vi "FPGA Target Approach RetractionA2copyAidan.vi"() -> ()   [LabVIEW 2012]
uses:
  <vilib>/rvi/FXPMathLib/basic elements/FxpIntAccumulator/subVIs/nifxpmath_IntAccumulator_SimConfig.ctl
  <vilib>/rvi/eio/common/nirviEmuTemplateMethod_errors.vi
  <vilib>/rvi/FXPMathLib/basic elements/FxpIntAccumulator/simVIs/DllFxpIntAccumulator_sub.vi
  <vilib>/rvi/interface/RandomDataEmulation/nirviRandomDataFPGAFIFO.vi
  <vilib>/rvi/interface/RandomDataEmulation/niFpgaRandomDataHandleErrors.vi
  <vilib>/rvi/Emulation/niFpgaSctlEmulationGetInTimedLoop.vi
  <vilib>/rvi/Emulation/niFpgaSctlEmulationGlobalWrite.vi
  <vilib>/eio/EIONode/EIONode.xnode
  <vilib>/rvi/FXPMathLib/basic elements/FxpIntAccumulator/XNode/nifxpmath_IntAccumulator.xnode
  <vilib>/rvi/Analysis/common/FxpNativeNode/niFpgaFxpNative.xnode
  <vilib>/rvi/Analysis/measure/butterworth/XNode/niFpgaButterworthFilter.xnode
  <vilib>/rvi/DataTransferAndStorage/Container/XNode/niFpgaContainer.xnode
  <vilib>/rvi/interface/RandomDataEmulation/nirviRandomDataFpgaReadWriteTemplate.vi
panel:
  in  "Feedback?":bool
  in  "Integral Constant":i16
  out "SummationFeedback":fxp<+/-,16,16>
  in  "Porportional Constant":i16
  out "Numeric 4":i32
  out "Numeric 3":i32
  out "Numeric 2":i32
  out "Numeric":i32
  in  "TF in Air":i32
  in  "Approach Minimum":i32
  in  "Approach Setpoint":i32
  in  "Fast Approach Offset":i32
  out "SummationfA":fxp<+/-,64,38>
  in  "Fine Approach Speed":fxp<+,64,38>
  out "SummationfR":fxp<+/-,64,38>
  in  "Fine Retraction Speed":fxp<+,64,38>
  out "SummationFA":fxp<+/-,64,38>
  out "Test Case Number Indicator":i16
  in  "Fast Approach Speed":fxp<+,64,38>
  in  "Approach":bool
  out "SummationFR":fxp<+/-,64,38>
  in  "Data Acquisition Rate":i16
  out "Ticks":i16
  out "HV/10":i16
  out "Tuning Fork Signal":fxp<+/-,24,17>
  in  "Fast Retraction Speed":fxp<+,64,38>
  out "Z Fine Indicator":fxp<+/-,40,30>
  out "Counter Indicator":fxp<+/-,64,32>
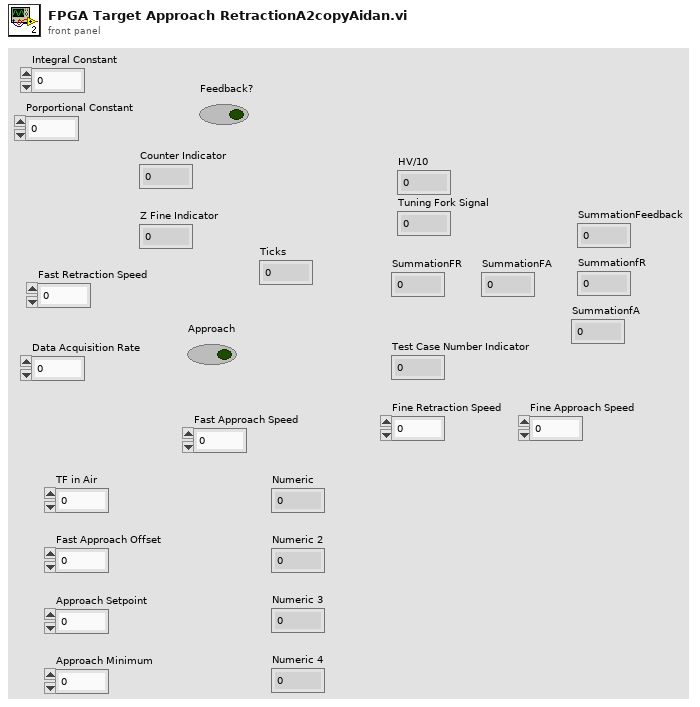
[diagram p1: front panel]
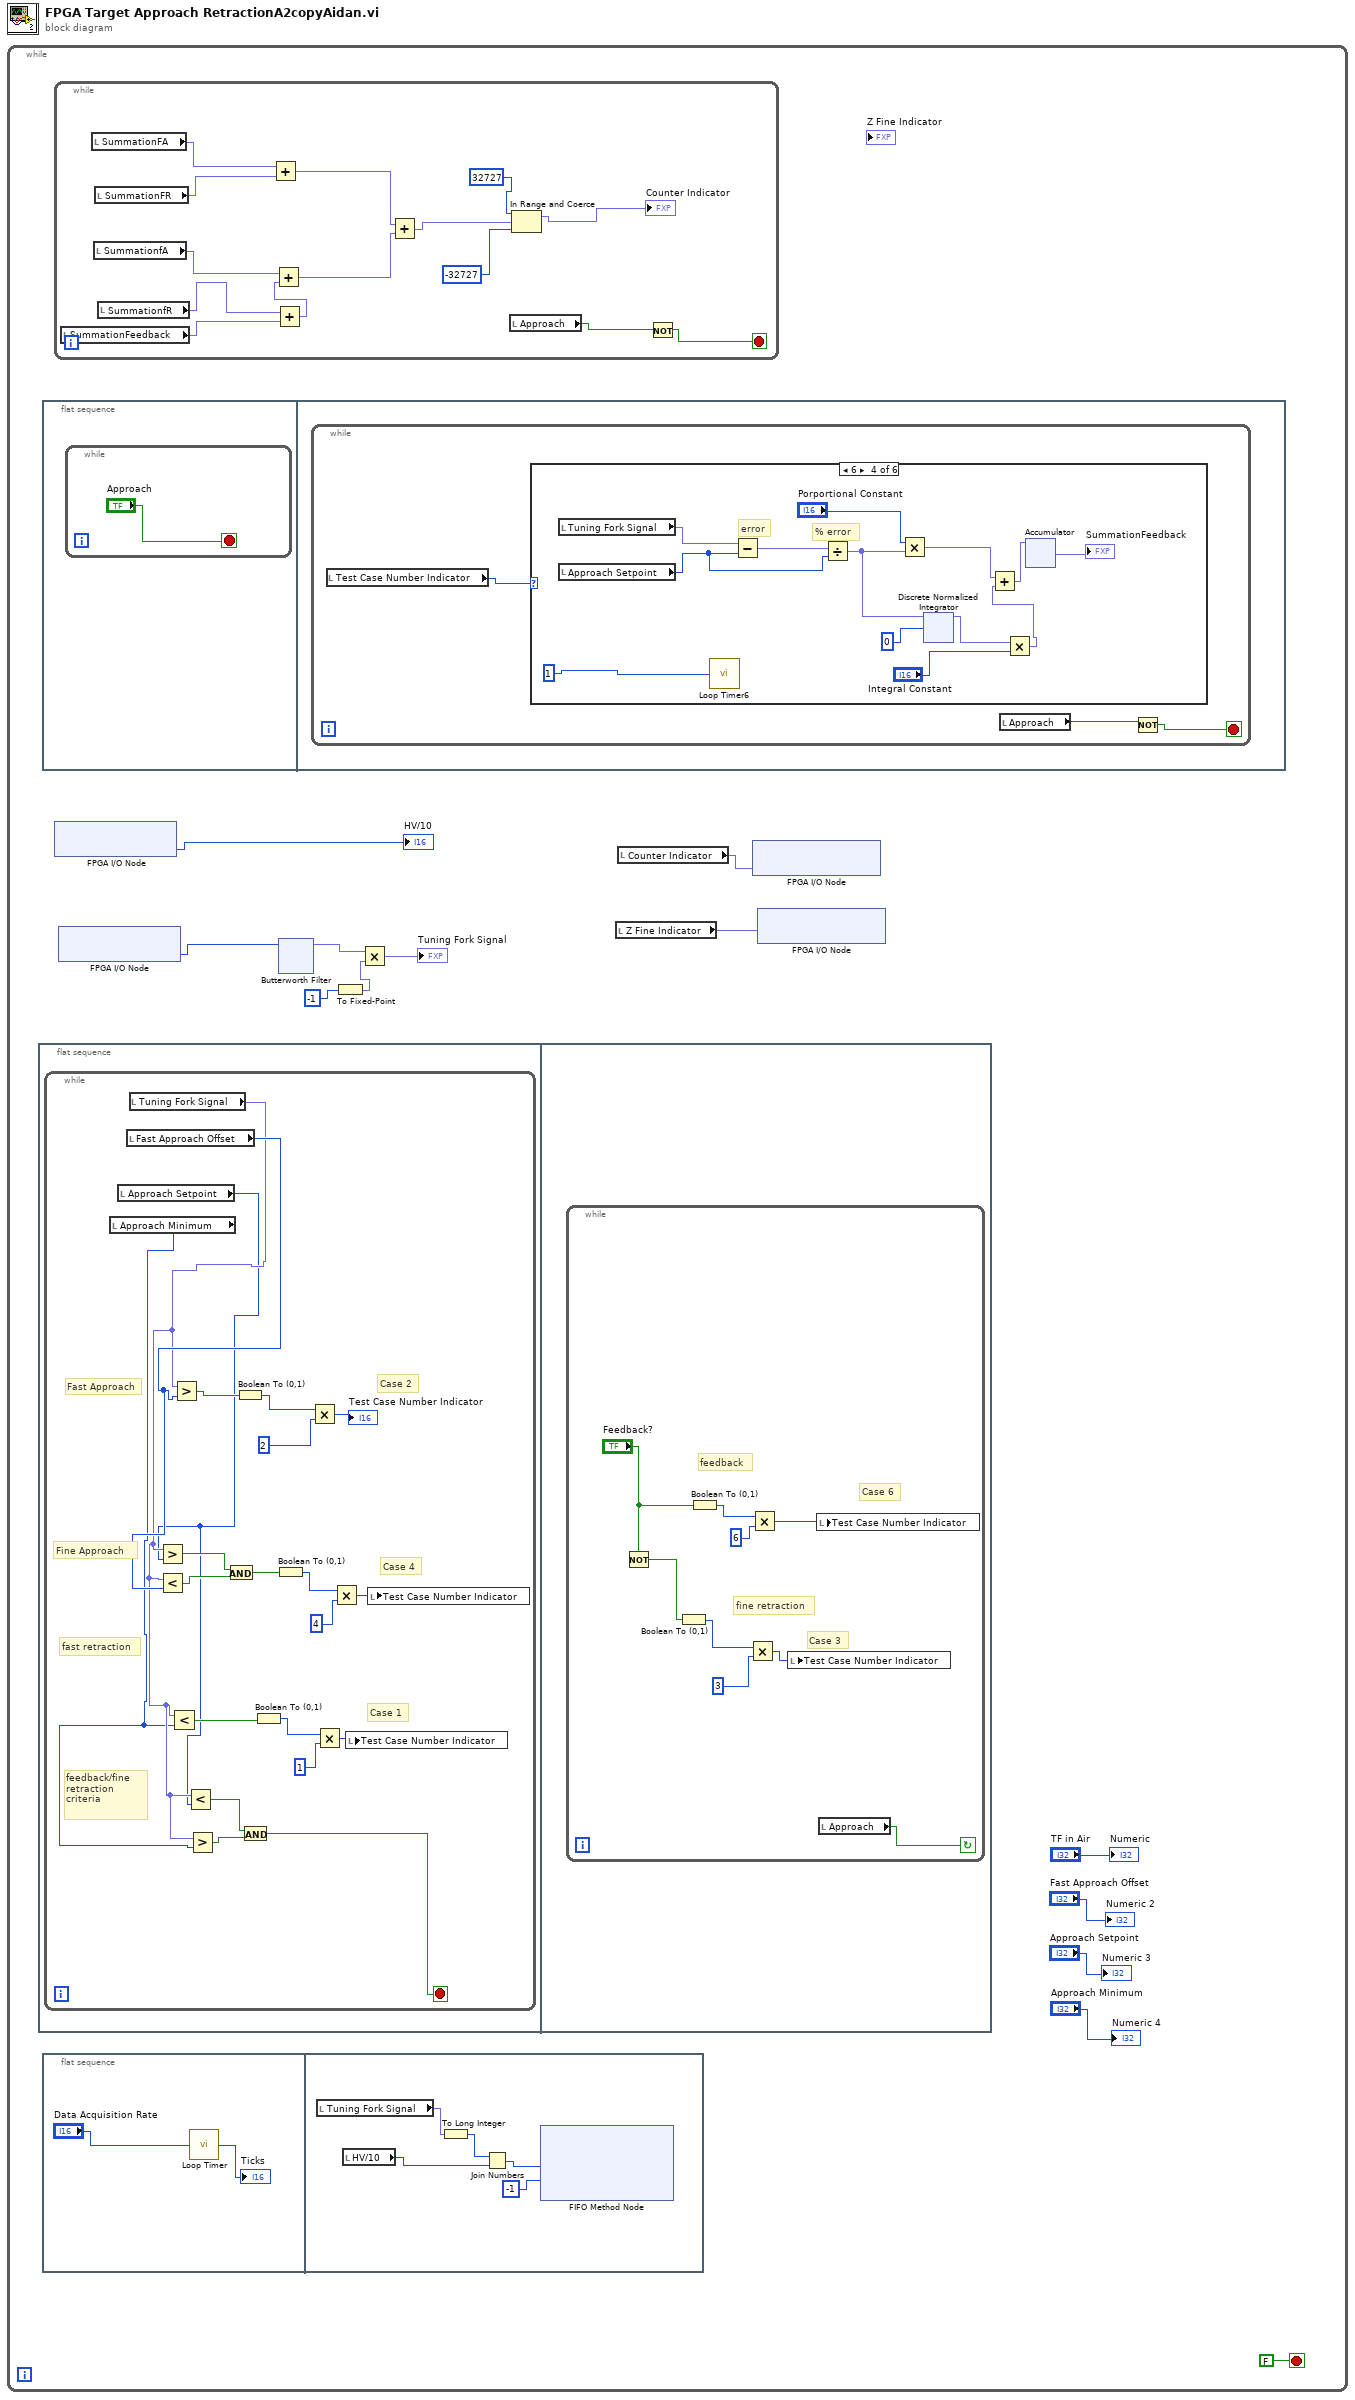
[diagram p0: block diagram]
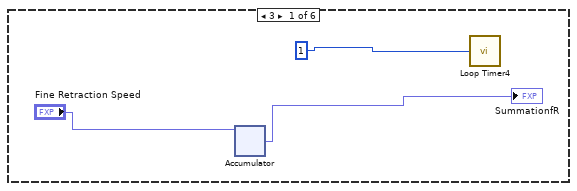
[diagram p2: hidden frame]
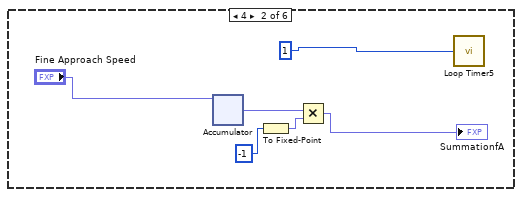
[diagram p3: hidden frame]
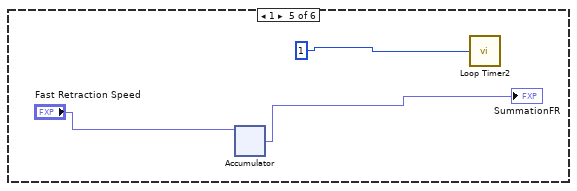
[diagram p5: hidden frame]
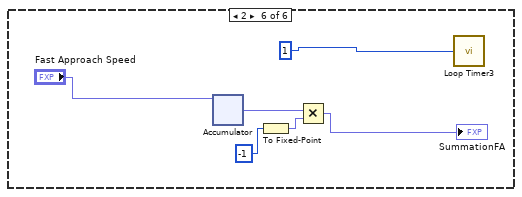
[diagram p6: hidden frame]
diagram:
  n1 = while {
    stop <- FALSE stop-if-true
    n2 = flat-sequence {
      frame #0 {
        n3 = while {
          stop <- w229 stop-if-true
          # "Case 1"
          # "Case 4"
          # "Case 2"
          # "feedback/fine retraction criteria"
          # "fast retraction"
          # "Fine Approach"
          # "Fast Approach"
          n4 = local read "Approach Minimum"() -> (w233:i32)
          n5 = local read "Approach Setpoint"() -> (w232:i32)
          n6 = local read "Fast Approach Offset"() -> (w238:i32)
          n7 = local read "Tuning Fork Signal"() -> (w234:fxp<+/-,24,17>)
          n8 = Greater?(x=w234, y=w232) -> (0:w243:bool)
          n9 = Less?(x=w234, y=w238) -> (x < y?=w242:bool)
          n10 = Less?(x=w234, y=w233) -> (x < y?=w235:bool)
          n11 = Greater?(x=w234, y=w238) -> (0:w241:bool)
          n12 = Less?(x=w234, y=w232) -> (x < y?=w231:bool)
          n13 = Greater?(x=w234, y=w233) -> (0:w230:bool)
          n14 = And(x=w243, y=w242) -> (x .and. y?=w246:bool)
          n15 = Boolean To (0,1)(Boolean=w241) -> (0, 1=w240:i16)
          n16 = And(x=w231, y=w230) -> (x .and. y?=w229:bool)
          n17 = Boolean To (0,1)(Boolean=w235) -> (0, 1=w236:i16)
          n18 = Boolean To (0,1)(Boolean=w246) -> (0, 1=w245:i16)
          n19 = Multiply(x=w240, y=i16 2) -> (x*y=→"Test Case Number Indicator":i16)
          n20 = Multiply(x=w236, y=i16 1) -> (x*y=w227:i16)
          n21 = Multiply(x=w245, y=i16 4) -> (x*y=w226:i16)
          n22 = local write "Test Case Number Indicator"(w227) -> ()
          n23 = local write "Test Case Number Indicator"(w226) -> ()
        }
      }
      frame #1 {
        n24 = while {
          stop <- w247 continue-if-true
          # "Case 6"
          # "Case 3"
          # "feedback"
          # "fine retraction"
          n25 = Not(x="Feedback?") -> (.not. x?=w250:bool)
          n26 = Boolean To (0,1)(Boolean=w250) -> (0, 1=w249:i16)
          n27 = Boolean To (0,1)(Boolean="Feedback?") -> (0, 1=w252:i16)
          n28 = Multiply(x=w249, y=i16 3) -> (x*y=w255:i16)
          n29 = Multiply(x=w252, y=i16 6) -> (x*y=w254:i16)
          n30 = local write "Test Case Number Indicator"(w255) -> ()
          n31 = local write "Test Case Number Indicator"(w254) -> ()
          n32 = local read "Approach"() -> (w247:bool)
        }
      }
    }
    n33 = flat-sequence {
      frame #0 {
        n34 = while {
          stop <- "Approach" stop-if-true
        }
      }
      frame #1 {
        n35 = while {
          stop <- w30 stop-if-true
          n36 = local read "Test Case Number Indicator"() -> (w29:i16)
          n37 = case shown="6" w29 {
            frame 3 {
              n38 = xnode "Accumulator"("x"="Fine Retraction Speed") -> ("s"=→"SummationfR":fxp<+,64,38>)  [unwired: 4 in, 1 out]
              n39 = call "Loop Timer4"("Count(uSec)"=i16 1) -> ()  [unwired: 1 out]
            }
            frame 4 {
              n40 = xnode "Accumulator"("x"="Fine Approach Speed") -> ("s"=w66:fxp<+,64,38>)  [unwired: 4 in, 1 out]
              n41 = To Fixed-Point(number=i16 -1) -> (fixed-point=w64:fxp<+/-,16,16>)  [unwired: 1 in]
              n42 = Multiply(x=w66, y=w64) -> (x*y=→"SummationfA":fxp<+/-,64,54>)
              n43 = call "Loop Timer5"("Count(uSec)"=i16 1) -> ()  [unwired: 1 out]
            }
            frame 5, Default {
            }
            frame 6 {
              # "% error"
              # "error"
              n44 = local read "Tuning Fork Signal"() -> (w107:fxp<+/-,24,17>)
              n45 = local read "Approach Setpoint"() -> (w105:i32)
              n46 = call "Loop Timer6"("Count(uSec)"=i16 1) -> ()  [unwired: 1 out]
              n47 = Subtract(x=w107, y=w105) -> (x-y=w106:fxp<+/-,40,33>)
              n48 = Divide(x=w106, y=w105) -> (x/y=w101:fxp<+/-,64,33>)
              n49 = Multiply(x="Porportional Constant", y=w101) -> (x*y=w97:fxp<+/-,64,49>)
              n50 = xnode ("Discrete Normalized Integrator")("initial condition"=i16 0, "input"=w101) -> ("output"=w99:fxp<+/-,64,49>)  [unwired: 1 in]
              n51 = Multiply(x=w99, y="Integral Constant") -> (x*y=w98:fxp<+/-,64,65>)
              n52 = Add(x=w97, y=w98) -> (x+y=w96:fxp<+/-,64,66>)
              n53 = xnode "Accumulator"("x"=w96) -> ("s"=→"SummationFeedback":fxp<+/-,64,66>)  [unwired: 4 in, 1 out]
            }
            frame 1 {
              n54 = xnode "Accumulator"("x"="Fast Retraction Speed") -> ("s"=→"SummationFR":fxp<+,64,38>)  [unwired: 4 in, 1 out]
              n55 = call "Loop Timer2"("Count(uSec)"=i16 1) -> ()  [unwired: 1 out]
            }
            frame 2 {
              n56 = xnode "Accumulator"("x"="Fast Approach Speed") -> ("s"=w180:fxp<+,64,38>)  [unwired: 4 in, 1 out]
              n57 = To Fixed-Point(number=i16 -1) -> (fixed-point=w182:fxp<+/-,16,16>)  [unwired: 1 in]
              n58 = Multiply(x=w180, y=w182) -> (x*y=→"SummationFA":fxp<+/-,64,54>)
              n59 = call "Loop Timer3"("Count(uSec)"=i16 1) -> ()  [unwired: 1 out]
            }
          }
          n60 = local read "Approach"() -> (w31:bool)
          n61 = Not(x=w31) -> (.not. x?=w30:bool)
        }
      }
    }
    n62 = flat-sequence {
      frame #0 {
        n63 = call "Loop Timer"("Count(uSec)"="Data Acquisition Rate") -> ("Tick Count(uSec)"=→"Ticks":u32)
      }
      frame #1 {
        n64 = local read "Tuning Fork Signal"() -> (w225:fxp<+/-,24,17>)
        n65 = local read "HV/10"() -> (w224:i16)
        n66 = To Long Integer(number=w225) -> (32bit integer=w223:i32)
        n67 = Join Numbers(hi=w223, lo=w224) -> ((hi.lo)=w222:u64)
        n68 = xnode ("FIFO Method Node")("Element"=w222, "Timeout"=i16 -1) -> ()  [unwired: 1 in, 2 out]
      }
    }
    n69 = while {
      stop <- w19 stop-if-true
      n70 = local read "SummationFeedback"() -> (w17:fxp<+/-,16,16>)
      n71 = local read "SummationFA"() -> (w27:fxp<+/-,64,38>)
      n72 = local read "SummationfA"() -> (w25:fxp<+/-,64,38>)
      n73 = local read "SummationFR"() -> (w26:fxp<+/-,64,38>)
      n74 = local read "SummationfR"() -> (w18:fxp<+/-,64,38>)
      n75 = Add(x=w27, y=w26) -> (x+y=w24:fxp<+/-,64,39>)
      n76 = Add(x=w18, y=w17) -> (x+y=w15:fxp<+/-,64,39>)
      n77 = Add(x=w25, y=w15) -> (x+y=w16:fxp<+/-,64,40>)
      n78 = Add(x=w24, y=w16) -> (x+y=w23:fxp<+/-,64,41>)
      n79 = local read "Approach"() -> (w20:bool)
      n80 = In Range and Coerce(upper limit=i16 32727, x=w23, lower limit=i16 -32727) -> (coerced(x)=→"Counter Indicator":fxp<+/-,64,41>)  [unwired: 1 out]
      n81 = Not(x=w20) -> (.not. x?=w19:bool)
    }
    n82 = xnode "FPGA I/O Node"() -> ("Connector0/AI6"=→"HV/10":i16)  [unwired: 1 in, 1 out]
    n83 = xnode "FPGA I/O Node"() -> ("Connector0/AI7"=w3:i16)  [unwired: 1 in, 1 out]
    n84 = xnode "Butterworth Filter"("input data"=w3) -> ("output data"=w7:fxp<+/-,20,20>)  [unwired: 2 in]
    n85 = To Fixed-Point(number=i16 -1) -> (fixed-point=w6:fxp<+/-,16,16>)  [unwired: 1 in]
    n86 = Multiply(x=w7, y=w6) -> (x*y=→"Tuning Fork Signal":fxp<+/-,36,36>)
    n87 = local read "Z Fine Indicator"() -> (w1:fxp<+/-,40,30>)
    n88 = local read "Counter Indicator"() -> (w2:fxp<+/-,64,32>)
    n89 = xnode "FPGA I/O Node"("Connector0/AO7"=w2) -> ()  [unwired: 1 in, 1 out]
    n90 = xnode "FPGA I/O Node"("Connector0/AO2"=w1) -> ()  [unwired: 1 in, 1 out]
    "Numeric" <- "TF in Air"
    "Numeric 2" <- "Fast Approach Offset"
    "Numeric 3" <- "Approach Setpoint"
    "Numeric 4" <- "Approach Minimum"
  }
